vi "Read Config v1.1.vi"(8 "error in":errorcluster, 11 "file path":path) -> (0 "error out":errorcluster, 2 "All Para":cluster{"Auto Para":T1, "General Para 2":T2}={"Auto Para"={"Agitator Delays"=[250, 600], "TF Delays"=[400, 800, 2, 8000], "Insertion Delays"=[100, 400], "Cutting Delays"=[150, 250, 50], "PF Delays"=[300, 8000], "Measur. Delays"=[200.0, 188.9, 1.0], "Reject Delays"=[500], "BF Delays"=[1000, 1000]}, "General Para 2"={"Max. Cons."=5.0, "Offset 1"=0.0, "Offset 2"=0.0, "Offset 3"=0.0, "Offset 4"=-0.6, "OutputPause"=500.0, "RejectPause"=500.0}} {"General Para 2"."Offset 4" format="%.2f"; "General Para 2"."Offset 3" format="%.2f"; "General Para 2"."Offset 2" format="%.2f"; "General Para 2"."Offset 1" format="%.2f"}, 3 "file path out":path, 5 "password":string)   [LabVIEW 2017]
doc: "v1.0:\nRead 2WR Motor Bencg or not."
uses:
  RT/Controls/Auto Delays.ctl
  Controls/General Para.ctl
  <vilib>/Utility/config.llb/Read Key (Double).vi
  <vilib>/Utility/config.llb/Read Key (String).vi
  <vilib>/Utility/config.llb/NI_LVConfig.lvlib
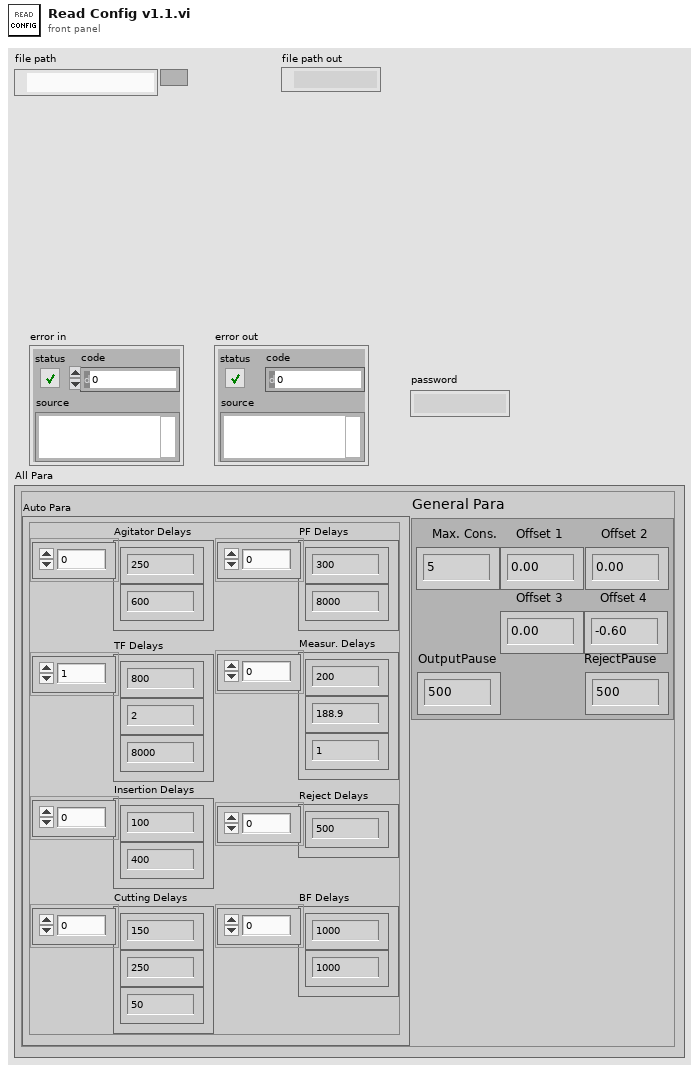
[diagram p1: front panel]
types:
  T1 = typedef "Auto Delays.ctl" = cluster{"Agitator Delays":u32[], "TF Delays":u32[], "Insertion Delays":u32[], "Cutting Delays":u32[], "PF Delays":u32[], "Measur. Delays":dbl[], "Reject Delays":u32[], "BF Delays":u32[]}
  T2 = typedef "General Para.ctl" = cluster{"Max. Cons.":dbl, "Offset 1":dbl, "Offset 2":dbl, "Offset 3":dbl, "Offset 4":dbl, "OutputPause":dbl, "RejectPause":dbl}
  T3 = typedef "NI_LVConfig.lvlib/Config Data RefNum.ctl" = refnum<k1>
  T4 = cluster{"[0]":dbl, "[1]":dbl, "[2]":dbl, "[3]":dbl, "[4]":dbl, "[5]":dbl, "[6]":dbl}
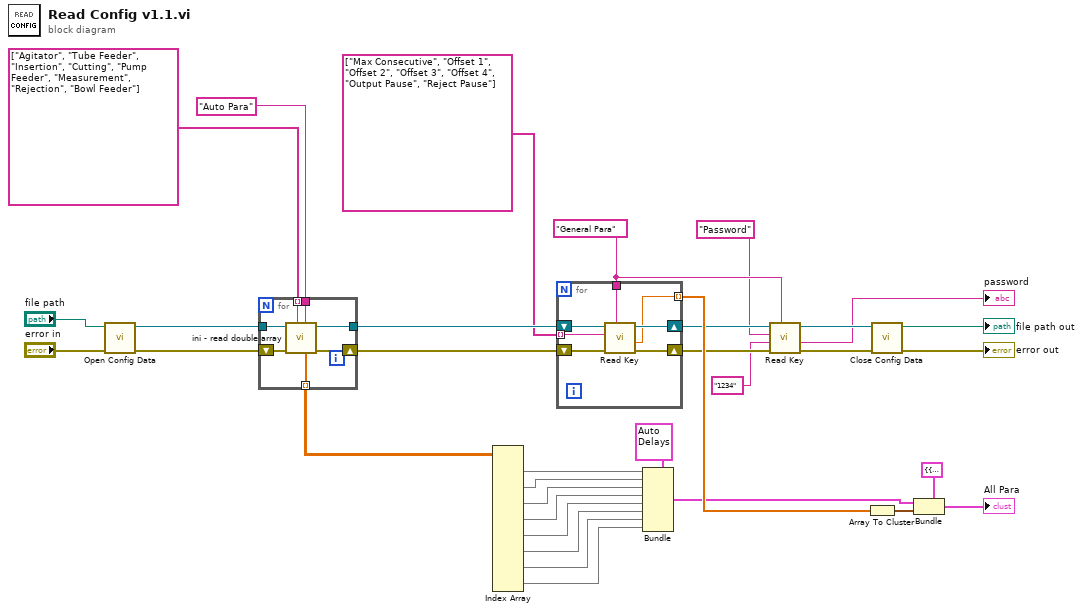
[diagram p0: block diagram]
diagram:
  w4 = "General Para" ("section")
  n1 = call <vilib>:"Open Config Data.vi"("error in (no error)"="error in", "configuration file path"="file path") -> ("error out"=w25:errorcluster, "refnum"=w26:T3)  [unwired: 7 in, 1 out]
  n2 = for {
    tunnel: w26 -> [w41]
    tunnel: "Auto Para" ("section") -> [w37]
    tunnel: string[] ["Agitator", "Tube Feeder", "Insertion", "Cutting", "Pump Feeder", "Measurement", "Rejection", "Bowl Feeder"] -> [w36] mode=indexing
    tunnel: [w38] -> w29
    shift-right: [w39] -> w28
    shift-left: w25 -> [w40]
    tunnel: [w35] -> w19 mode=indexing
    n3 = call "ini - read double array.vi"("section"=w37, "key"=w36, "error in"=w40, "refnum in"=w41) -> ("error out"=w39:errorcluster, "refnum out"=w38:T3, "double array"=w35:dbl[])  [unwired: 5 in]
  }
  n4 = Index Array(array=w19) -> (element #1=w18:dbl[], element #2=w17:dbl[], element #3=w16:dbl[], element #4=w15:dbl[], element #5=w14:dbl[], element #6=w13:dbl[], element #7=w12:dbl[], element #8=w11:dbl[])  [unwired: 16 in]
  n5 = for {
    tunnel: w4 -> [w46]
    shift-right: [w48] -> w6
    shift-left: w29 -> [w45]
    shift-right: [w47] -> w8
    shift-left: w28 -> [w44]
    tunnel: string[] ["Max Consecutive", "Offset 1", "Offset 2", "Offset 3", "Offset 4", "Output Pause", "Reject Pause"] -> [w43] mode=indexing
    tunnel: [w42] -> w21 mode=indexing
    n6 = call-poly <vilib>:"Read Key.vi"("section"=w46, "error in (no error)"=w44, "key"=w43, "refnum"=w45) -> ("error out"=w47:errorcluster, "value"=w42:dbl, "refnum out"=w48:T3)  [unwired: 4 in, 1 out]
  }
  n7 = Bundle(cluster=T1 {"Agitator Delays"=[250, 600], "TF Delays"=[400, 800, 2, 8000], "Insertion Delays"=[100, 400], "Cutting Delays"=[150, 250, 50], "PF Delays"=[300, 8000], "Measur. Delays"=[200.0, 188.9, 1.0], "Reject Delays"=[500], "BF Delays"=[1000, 1000]} ("Auto Para"), "Agitator Delays"=w18, "TF Delays"=w17, "Insertion Delays"=w16, "Cutting Delays"=w15, "PF Delays"=w14, "Measur. Delays"=w13, "Reject Delays"=w12, "BF Delays"=w11) -> (w10:T1)
  n8 = call-poly <vilib>:"Read Key.vi"("section"=w4, "error in (no error)"=w8, "default value"="1234", "key"="Password", "refnum"=w6) -> ("error out"=w7:errorcluster, "value"=→"password":string, "refnum out"=w5:T3)  [unwired: 3 in, 1 out]
  n9 = Array To Cluster(array=w21) -> (cluster=w22:T4)
  n10 = call <vilib>:"Close Config Data.vi"("error in (no error)"=w7, "refnum"=w5) -> ("error out"=→"error out":errorcluster, "file path"=→"file path out":path)  [unwired: 8 in]
  n11 = Bundle(cluster=cluster{"Auto Para":T1, "General Para 2":T2} {"Auto Para"={"Agitator Delays"=[250, 600], "TF Delays"=[400, 800, 2, 8000], "Insertion Delays"=[100, 400], "Cutting Delays"=[150, 250, 50], "PF Delays"=[300, 8000], "Measur. Delays"=[200.0, 188.9, 1.0], "Reject Delays"=[500], "BF Delays"=[1000, 1000]}, "General Para 2"={"Max. Cons."=5.0, "Offset 1"=0.0, "Offset 2"=0.0, "Offset 3"=0.0, "Offset 4"=-0.6, "OutputPause"=500.0, "RejectPause"=500.0}} ("All Para"), "Auto Para"=w10, "General Para 2"=w22) -> (→"All Para":cluster{"Auto Para":T1, "General Para 2":T2})
